vi "Read Vacuum.vi"(8 "error in":errorcluster, 11 "TSI 3010 in":refnum<class "TSI 3010.lvclass">) -> (0 "error out":errorcluster, 2 "Vacuum":u32, 3 "TSI 3010 out":refnum<class "TSI 3010.lvclass">)   [LabVIEW 2014, in "TSI 3010.lvclass"]
uses:
  TSI 3010.lvclass
  Controls/Vacuum.ctl
  CPC.lvclass/CPC.ctl
  Accessors/Read Session Handle.vi
  Accessors/Write Session Handle.vi
  reusable/Session APIs/Serial/Public/Get Data/Get String.vi
  reusable/Session APIs/Serial/Serial Session.lvclass
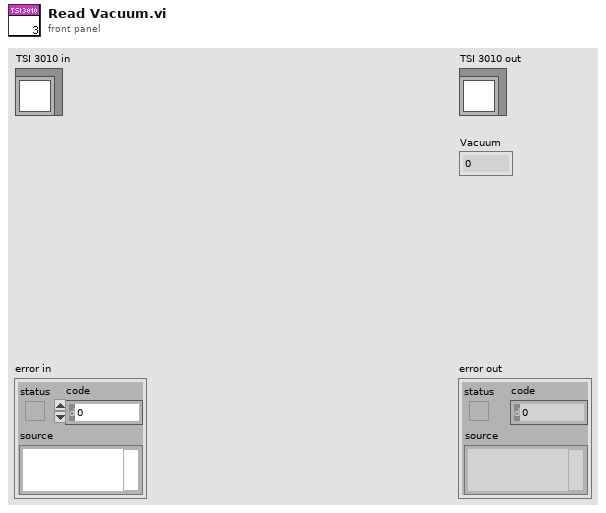
[diagram p1: front panel]
types:
  T1 = typedef "TSI 3010.lvclass/Vacuum.ctl" = enum16{"LOVAC", "VAC"}
  T2 = typedef "Serial Session.lvclass/Session Handle.ctl" = refnum<data-value>
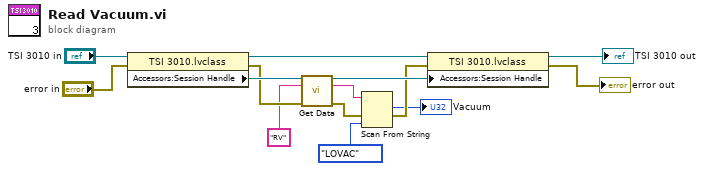
[diagram p0: block diagram]
diagram:
  n1 = property class="TSI 3010.lvclass"(reference="TSI 3010 in", error in="error in") -> (reference out=w10:refnum<class "TSI 3010.lvclass">, error out=w11:errorcluster, "Accessors:Session Handle"=w12:T2)
  n2 = call-poly "Get Data.vi"("Session Handle in"=w12, "CMD"="RV", "error in"=w11) -> ("Session Handle out"=w9:T2, "DataOut"=w4:string, "error out"=w3:errorcluster)  [unwired: 10 in]
  n3 = Scan From String(input string=w4, error in=w3, default 1=Vacuum."LOVAC" ("vacuum")) -> (offset past scan=→"Vacuum":u32, error out=w2:errorcluster)  [unwired: 3 in, 1 out]
  n4 = property class="TSI 3010.lvclass"(reference=w10, error in=w2, "Accessors:Session Handle"=w9) -> (reference out=→"TSI 3010 out":refnum<class "TSI 3010.lvclass">, error out=→"error out":errorcluster)
